vi "MGI Spline Interpolant with Derivative.vi"(0 "x[]":dbl[](array[numeric]) format="%.2f", 1 "y[]":dbl[](array[numeric]) format="%.2f") -> (2 "Interpolant[]":dbl[](array[numeric]) format="%.2f", 3 "First Derivative[]":dbl[](array[numeric]) format="%.2f", 4 "error":i32)   [LabVIEW 2016]
doc: "Calculate the Spline Interpolant and also the first derivative of the spline curve.\n\nAuthored by David A. Moore\nsupport@mooregoodideas.com\nwww.mooregoodideas.com\n\nCopyright (c) 2010, Moore Good Ideas, Inc.\n\nAll rights reserved.\n\nRedistribution and use in source and binary forms, with or without modification, are permitted provided that the following conditions are met:\n\n * Redistributions of source code must retain the above copyright notice, this list of conditions and the following disclaimer.\n * Redistributions in binary form must reproduce the above copyright notice, this list of conditions and the following disclaimer in the documentation and/or other materials provided with the distribution.\n * Neither the name of Moore Good Ideas, Inc. nor the names of its contributors may be used to endorse or promote products derived from this software without specific prior written permission.\n\nTHIS SOFTWARE IS PROVIDED BY THE COPYRIGHT HOLDERS AND CONTRIBUTORS \"AS IS\" AND ANY EXPRESS OR IMPLIED WARRANTIES, INCLUDING, BUT NOT LIMITED TO, THE IMPLIED WARRANTIES OF MERCHANTABILITY AND FITNESS FOR A PARTICULAR PURPOSE ARE DISCLAIMED. IN NO EVENT SHALL THE COPYRIGHT OWNER OR CONTRIBUTORS BE LIABLE FOR ANY DIRECT, INDIRECT, INCIDENTAL, SPECIAL, EXEMPLARY, OR CONSEQUENTIAL DAMAGES (INCLUDING, BUT NOT LIMITED TO, PROCUREMENT OF SUBSTITUTE GOODS OR SERVICES; LOSS OF USE, DATA, OR PROFITS; OR BUSINESS INTERRUPTION) HOWEVER CAUSED AND ON ANY THEORY OF LIABILITY, WHETHER IN CONTRACT, STRICT LIABILITY, OR TORT (INCLUDING NEGLIGENCE OR OTHERWISE) ARISING IN ANY WAY OUT OF THE USE OF THIS SOFTWARE, EVEN IF ADVISED OF THE POSSIBILITY OF SUCH DAMAGE."
uses:
  <vilib>/Analysis/NI_AALPro.lvlib
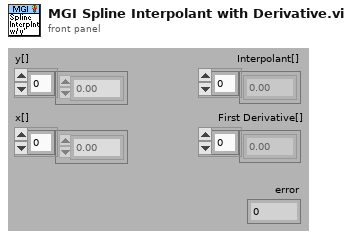
[diagram p1: front panel]
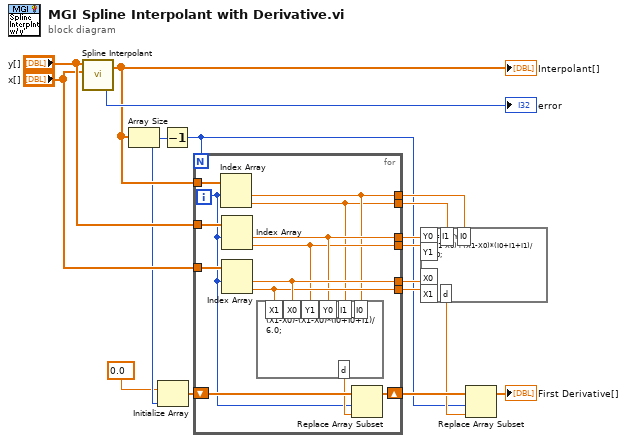
[diagram p0: block diagram]
diagram:
  n1 = call <vilib>:"Spline Interpolant.vi"("X"="x[]", "Y"="y[]") -> ("error"=→"error":i32, "Interpolant"=w14:dbl[])  [unwired: 2 in]
  "Interpolant[]" <- w14
  n2 = Array Size(array=w14) -> (size(s)=w6:i32)
  n3 = Initialize Array(0.0, w6) -> (w7:dbl[])
  n4 = Decrement(x=w6) -> (x-1=w1:i32)
  n5 = for {
    N: w1 -> [_]
    tunnel: "y[]" -> [w30]
    tunnel: "x[]" -> [w29]
    tunnel: w14 -> [w28]
    tunnel: [w23] -> w8
    tunnel: [w22] -> w9
    tunnel: [w25] -> w10
    tunnel: [w24] -> w11
    tunnel: [w27] -> w12
    tunnel: [w26] -> w13
    shift-right: [w21] -> w4
    shift-left: w7 -> [w20]
    i -> [w18]
    n6 = Index Array(array=w28, index #1=w18) -> (element #1=w23:dbl, element #2=w22:dbl)  [unwired: 1 in]
    n7 = Index Array(array=w30, index #1=w18) -> (element #1=w25:dbl, element #2=w24:dbl)  [unwired: 1 in]
    n8 = Index Array(array=w29, index #1=w18) -> (element #1=w27:dbl, element #2=w26:dbl)  [unwired: 1 in]
    n9 = formula code="d=(Y1-Y0)/(X1-X0)-(X1-X0)*(I0+I0+I1)/6.0;"("X0"=w27, "X1"=w26, "Y0"=w25, "Y1"=w24, "I0"=w23, "I1"=w22) -> ("d"=w19:dbl)
    n10 = Replace Array Subset(array=w20, new element=w19, index=w18) -> (w21:dbl[])
  }
  n11 = formula code="d=(Y1-Y0)/(X1-X0)+(X1-X0)*(I0+I1+I1)/6.0;"("X0"=w12, "X1"=w13, "Y0"=w10, "Y1"=w11, "I0"=w8, "I1"=w9) -> ("d"=w3:dbl)
  n12 = Replace Array Subset(array=w4, new element=w3, index=w1) -> (→"First Derivative[]":dbl[])
